vi "LVM Fixer.vi"(8 "Error In":errorcluster, 10 "Folder":path=path "E:/LabVIEW/Data/Test Data/Subj-Austin_Trial-1_Condition-None.lvm" caption="Filename") -> (0 "Error Out":errorcluster)   [LabVIEW 2020]
uses:
  <vilib>/express/express shared/transition.llb/Dynamic To Waveform Array.vi
  <vilib>/express/express signal manip/GetorSetDDTAttributes/Shared VIs/XDimension conversion.vi
  <vilib>/express/express signal manip/GetorSetDDTAttributes/Shared VIs/XDimension Enum to String.vi
  <vilib>/express/express signal manip/GetorSetDDTAttributes/Shared VIs/TimeMode Enum to Boolean.vi
  <vilib>/express/express signal manip/GetorSetDDTAttributes/Set DDT Attributes/SetT0.vi
  <vilib>/express/express signal manip/GetorSetDDTAttributes/Set DDT Attributes/sub Set StartTimeStamp.vi
  <vilib>/express/express shared/transition.llb/Waveform Array To Dynamic.vi
  <vilib>/express/express signal manip/GetorSetDDTAttributes/Get DDT Attributes/Get DDT Properties.xnode
  <vilib>/express/express signal manip/GetorSetDDTAttributes/Shared VIs/TimeType.ctl
  <vilib>/express/express signal manip/GetorSetDDTAttributes/Shared VIs/XDimension.ctl
  <vilib>/express/express signal manip/GetorSetDDTAttributes/Set DDT Attributes/Set DDT Properties.xnode
  <vilib>/express/express signal manip/GetorSetDDTAttributes/Shared VIs/GetSetShared.lvlib
  <vilib>/express/express signal manip/GetorSetDDTAttributes/Set DDT Attributes/Set DDT Attributes.lvlib
panel:
  out "Total Rows Deleted":i32
  out "Display Table":string[][](table)
  out "Progress Bar":u8(slide) max=10 scale=0.9..27.0
  out "Number of Files Found":i32
  in  "Stop Button":bool
  out "Files Checked":i32
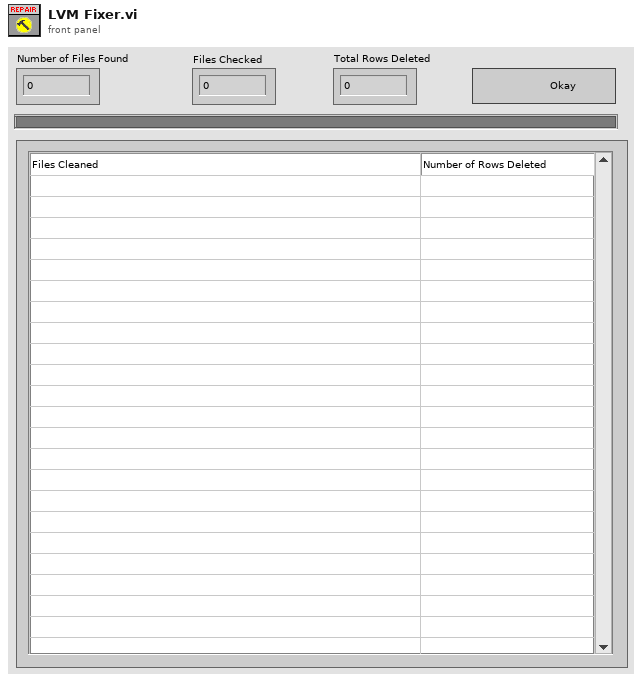
[diagram p1: front panel]
types:
  T1 = typedef "GetSetShared.lvlib/TimeType.ctl" = enum16{"Absolute", "Relative"}
  T2 = typedef "GetSetShared.lvlib/XDimension.ctl" = enum16{"No Unit [-]", "Time [sec]", "Frequency [Hz]"}
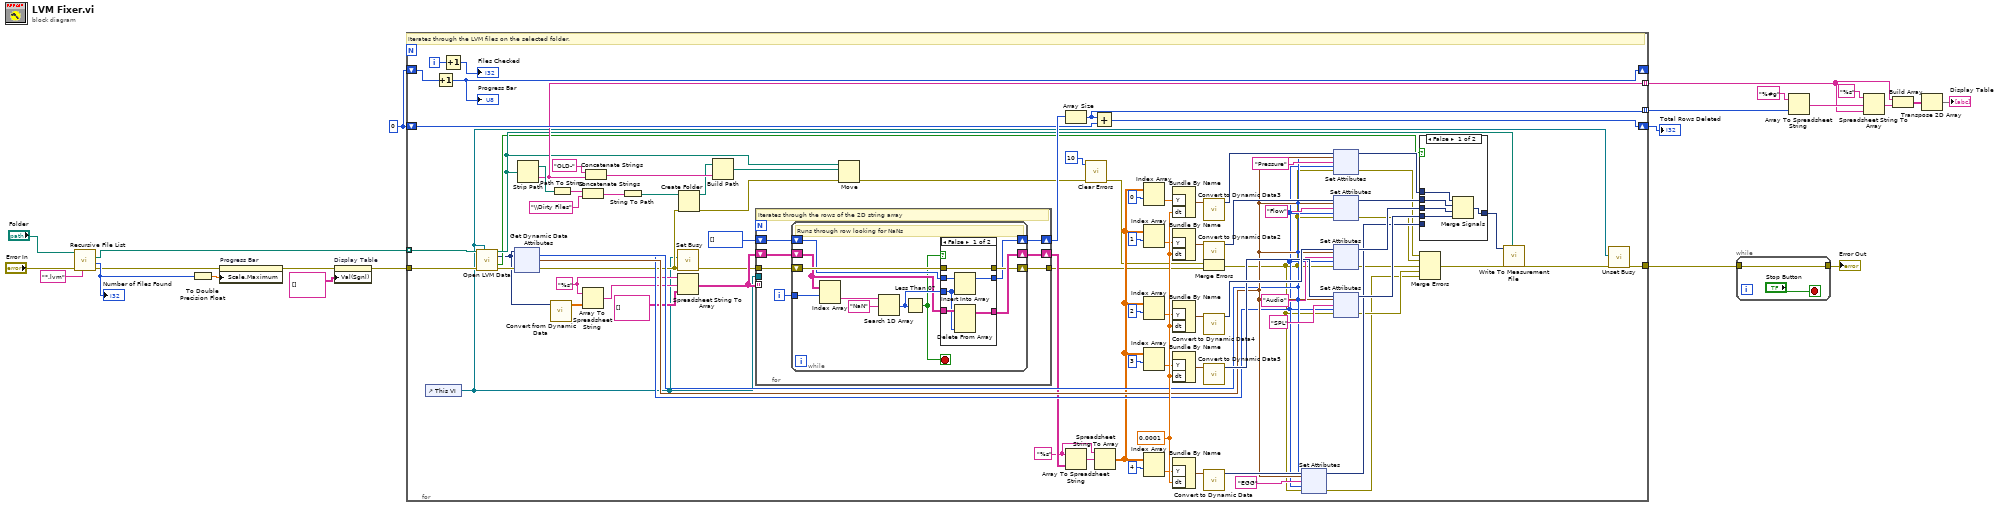
[diagram p0: block diagram]
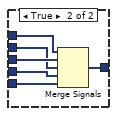
[diagram p3: hidden frame]
diagram:
  w3 = 0 ("x+1")
  n1 = call <vilib>:"Recursive File List.vi"("pattern"="*.lvm", "error in (no error)"="Error In", "Folder Path"="Folder") -> ("error out"=w11:errorcluster, "Number of Files"=w13:i32, "All Files in Dir"=w21:path[])  [unwired: 4 in, 2 out]
  "Number of Files Found" <- w13
  n2 = To Double Precision Float(number=w13) -> (double precision float=w12:dbl)
  n3 = property on="Progress Bar" class="Slide (strict)"(error in=w11, "Scale.Maximum"=w12) -> (error out=w6:errorcluster)  [unwired: 1 in, 1 out]
  n4 = property on="Display Table" class="Tbl (strict)"(error in=w6, "Val(Sgnl)"=string[][] [] ("Value (Signaling)")) -> (error out=w5:errorcluster)  [unwired: 1 in, 1 out]
  n5 = for {
    tunnel: w5 -> [w28]
    tunnel: [w87] -> w19
    tunnel: w21 -> [w27] mode=indexing
    tunnel: [w33] -> w15 mode=indexing
    tunnel: [w49] -> w14 mode=indexing
    shift-right: [w52] -> _
    shift-left: w3 -> [w53]
    shift-right: [w48] -> w2
    shift-left: w3 -> [w50]
    i -> [w56]
    w65 = "%s" ("format string")
    w70 = "%s" ("format string")
    w88 = 0.0001 ("dt")
    # "Iterates through the LVM files on the selected folder."
    n6 = control-ref of="This VI"() -> (w26:refnum<vi>)
    n7 = Increment(x=w53) -> (x+1=w52:i32)
    "Progress Bar" <- w52
    n8 = Increment(x=w56) -> (x+1=→"Files Checked":i32)
    n9 = call "Open LVM Data.vi"("Filename"=w27, "VI reference"=w26, "Error In"=w28) -> ("Filename Out"=w25:path, "All Data"=w23:dynamicdata, "EGG?"=w24:bool, "Error Out"=w29:errorcluster)  [unwired: 9 in]
    n10 = xnode "Get Dynamic Data Attributes"("Signals In"=w23, "error in"=w29) -> ("error out"=w38:errorcluster, "Time Mode"=w73:T1, "Timestamp"=w75:timestamp, "X Dimension"=w74:T2)  [unwired: 1 in, 2 out]
    n11 = Strip Path(path=w25) -> (stripped path=w46:path, name=w33:string)
    n12 = call "Convert from Dynamic Data"("Dynamic Data Type"=w23) -> ("Array"=w68:dbl[][])  [unwired: 3 in]
    n13 = Path To String(path=w46) -> (string=w45:string)
    n14 = Array To Spreadsheet String(array=w68, 3:w70) -> (spreadsheet string=w40:string)  [unwired: 1 in]
    n15 = Concatenate Strings(w45, "\\Dirty Files" ("string")) -> (w43:string)
    n16 = Concatenate Strings("OLD-" ("string"), w33) -> (w37:string)
    n17 = String To Path(string=w43) -> (path=w36:path)
    n18 = call <vilib>:"Set Busy.vi"("error in (no error)"=w38, "VI reference (current VI)"=w26) -> ("error out"=w54:errorcluster)  [unwired: 8 in, 1 out]
    n19 = Spreadsheet String To Array(format string=w70, spreadsheet string=w40, array type (2D Dbl)=string[][] []) -> (array=w58:string[][])  [unwired: 1 in]
    n20 = Create Folder(path (use dialog)=w36, error in=w38) -> (created path=w35:path, error out=w32:errorcluster)  [unwired: 1 in, 1 out]
    n21 = Build Path(base path=w35, name or relative path=w37) -> (appended path=w39:path)
    n22 = for {
      tunnel: [w112] -> w42
      tunnel: w54 -> [w111]
      shift-right: [w113] -> w51
      shift-left: i32[] [] -> [w114]
      tunnel: w26 -> [_]
      shift-right: [w115] -> w66
      shift-left: w58 -> [w110]
      tunnel: w58 -> [_] mode=indexing
      i -> [w109]
      # "Iterates through the rows of the 2D string array"
      n23 = while {
        shift-right: [w124] -> w115
        shift-left: w110 -> [w118]
        shift-right: [w122] -> w112
        shift-left: w111 -> [w123]
        shift-right: [w120] -> w113
        shift-left: w114 -> [w121]
        tunnel: w109 -> [w119]
        stop <- w116 stop-if-true
        # "Runs through row looking for NaNs"
        n24 = Index Array(array=w118, index (row)=w119) -> (element=w117:string[])  [unwired: 1 in]
        n25 = Search 1D Array(1D array=w117, element="NaN") -> (index of element=w125:i32)  [unwired: 1 in]
        n26 = Less Than 0?(x=w125) -> (x < 0?=w116:bool)
        n27 = case shown="False" w116 {
          tunnel: w125 -> [w127 _]
          tunnel: [w132 w135] -> w124
          tunnel: w118 -> [w131 w135]
          tunnel: w123 -> [w130 w134]
          tunnel: [w130 w134] -> w122
          tunnel: w121 -> [w129 w133]
          tunnel: [w128 w133] -> w120
          frame False {
            n28 = Insert Into Array(array=w129, new element=w127) -> (w128:i32[])  [unwired: 1 in]
            n29 = Delete From Array(array=w131, index (col)=w127) -> (array with subset deleted=w132:string[][])  [unwired: 2 in, 1 out]
          }
          frame True {
          }
        }
      }
    }
    n30 = Move(source path=w25, error in=w32, 10:w39) -> (error out=w31:errorcluster)  [unwired: 2 in, 2 out]
    n31 = Array Size(array=w51) -> (size(s)=w49:i32)
    n32 = Array To Spreadsheet String(array=w66, 3:w65) -> (spreadsheet string=w64:string)  [unwired: 1 in]
    n33 = call <vilib>:"Clear Errors.vi"("error in (no error)"=w31, "specific error code to clear (0: all)"=10) -> ("error out"=w30:errorcluster)  [unwired: 4 in, 1 out]
    n34 = Add(x=w49, y=w50) -> (x+y=w48:i32)
    n35 = Spreadsheet String To Array(format string=w65, spreadsheet string=w64) -> (array=w67:dbl[][])  [unwired: 2 in]
    n36 = Index Array(array=w67, index (row)=0) -> (element=w63:dbl[])  [unwired: 1 in]
    n37 = Index Array(array=w67, index (row)=1) -> (element=w62:dbl[])  [unwired: 1 in]
    n38 = Index Array(array=w67, index (row)=2) -> (element=w61:dbl[])  [unwired: 1 in]
    n39 = Index Array(array=w67, index (row)=3) -> (element=w60:dbl[])  [unwired: 1 in]
    n40 = Index Array(array=w67, index (row)=4) -> (element=w59:dbl[])  [unwired: 1 in]
    n41 = Bundle By Name("Y"=w63, "dt"=w88) -> (w93:waveform(dbl))  [unwired: 1 in]
    n42 = Bundle By Name("Y"=w62, "dt"=w88) -> (w92:waveform(dbl))  [unwired: 1 in]
    n43 = Bundle By Name("Y"=w61, "dt"=w88) -> (w89:waveform(dbl))  [unwired: 1 in]
    n44 = Bundle By Name("Y"=w60, "dt"=w88) -> (w90:waveform(dbl))  [unwired: 1 in]
    n45 = Bundle By Name("Y"=w59, "dt"=w88) -> (w91:waveform(dbl))  [unwired: 1 in]
    n46 = call "Convert to Dynamic Data3"("Waveform"=w93) -> ("Dynamic Data Type"=w105:dynamicdata)  [unwired: 3 in]
    n47 = call "Convert to Dynamic Data2"("Waveform"=w92) -> ("Dynamic Data Type"=w103:dynamicdata)  [unwired: 3 in]
    n48 = Merge Errors(w30, w42) -> (w41:errorcluster)
    n49 = call "Convert to Dynamic Data4"("Waveform"=w89) -> ("Dynamic Data Type"=w100:dynamicdata)  [unwired: 3 in]
    n50 = call "Convert to Dynamic Data5"("Waveform"=w90) -> ("Dynamic Data Type"=w98:dynamicdata)  [unwired: 3 in]
    n51 = call "Convert to Dynamic Data"("Waveform"=w91) -> ("Dynamic Data Type"=w97:dynamicdata)  [unwired: 3 in]
    n52 = xnode "Set Attributes"("Signals In"=w97, "error in"=w41, "Signal Name"="EGG", "Time Mode"=w73, "Timestamp"=w75, "X Dimension"=w74) -> ("Signals Out"=w95:dynamicdata, "error out"=w76:errorcluster)  [unwired: 2 in]
    n53 = xnode "Set Attributes"("Signals In"=w105, "error in"=w41, "Signal Name"="Pressure", "Time Mode"=w73, "Timestamp"=w75, "X Dimension"=w74) -> ("Signals Out"=w94:dynamicdata, "error out"=w80:errorcluster)  [unwired: 2 in]
    n54 = xnode "Set Attributes"("Signals In"=w103, "error in"=w41, "Signal Name"="Flow", "Time Mode"=w73, "Timestamp"=w75, "X Dimension"=w74) -> ("Signals Out"=w101:dynamicdata, "error out"=w79:errorcluster)  [unwired: 2 in]
    n55 = xnode "Set Attributes"("Signals In"=w100, "error in"=w41, "Signal Name"="Audio", "Time Mode"=w73, "Timestamp"=w75, "X Dimension"=w74) -> ("Signals Out"=w99:dynamicdata, "error out"=w78:errorcluster)  [unwired: 2 in]
    n56 = xnode "Set Attributes"("Signals In"=w98, "error in"=w41, "Signal Name"="SPL", "Time Mode"=w73, "Timestamp"=w75, "X Dimension"=w74) -> ("Signals Out"=w96:dynamicdata, "error out"=w77:errorcluster)  [unwired: 2 in]
    n57 = case shown="False" w24 {
      tunnel: [w321 w327] -> w72
      tunnel: w94 -> [w320 w326]
      tunnel: w101 -> [w319 w324]
      tunnel: w99 -> [w318 w325]
      tunnel: w96 -> [w317 w323]
      tunnel: w95 -> [_ w322]
      frame False {
        n58 = Merge Signals(w320, w319, w318, w317) -> (w321:dynamicdata)
      }
      frame True {
        n59 = Merge Signals(w326, w325, w324, w323, w322) -> (w327:dynamicdata)
      }
    }
    n60 = Merge Errors(w80, w79, w78, w77, w76) -> (w81:errorcluster)
    n61 = call "Write To Measurement File"("Signals"=w72, "error in (no error)"=w81, "Filename"=w25) -> ("error out"=w57:errorcluster)  [unwired: 14 in, 2 out]
    n62 = call <vilib>:"Unset Busy.vi"("error in (no error)"=w57, "VI reference (current VI)"=w26) -> ("error out"=w87:errorcluster)  [unwired: 9 in]
  }
  "Total Rows Deleted" <- w2
  n63 = while {
    tunnel: w19 -> [w328]
    tunnel: [w328] -> w9
    stop <- "Stop Button" stop-if-true
  }
  "Error Out" <- w9
  n64 = Array To Spreadsheet String(array=w14, 3:"%#g" ("format string")) -> (spreadsheet string=w16:string)  [unwired: 1 in]
  n65 = Spreadsheet String To Array(format string="%s", spreadsheet string=w16, array type (2D Dbl)=w15) -> (array=w17:string[])  [unwired: 1 in]
  n66 = Build Array(w15, w17) -> (w18:string[][])
  n67 = Transpose 2D Array(2D array=w18) -> (transposed array=→"Display Table":string[][])
